vi "tx_pduGen.vi"(5 "byte array":u8[](array[numeric])) -> (0 "packet bits length":i32, 2 "pdu":i32[](array[numeric]))   [LabVIEW 2014]
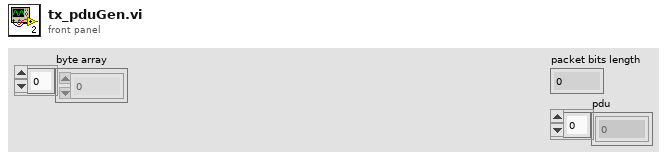
[diagram p1: front panel]
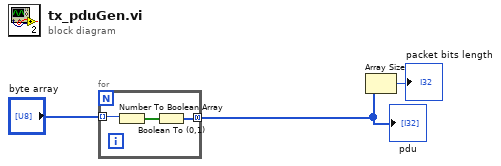
[diagram p0: block diagram]
diagram:
  n1 = for {
    tunnel: "byte array" -> [w6] mode=indexing
    tunnel: [w4] -> w1 mode=concatenating
    n2 = Number To Boolean Array(number=w6) -> (Boolean array=w5:bool[])
    n3 = Boolean To (0,1)(Boolean=w5) -> (0, 1=w4:i16[])
  }
  "pdu" <- w1
  n4 = Array Size(array=w1) -> (size(s)=→"packet bits length":i32)
